vi "test-Coordinate-System-Test4.vi"() -> (3 "All tests passed":bool)   [LabVIEW 2019]
uses:
  <vilib>/Rock Robotics/WPI/ThirdParty/JAS_Junk/TrajLib/VI/CoordAxis_N.vi
  <vilib>/Rock Robotics/WPI/ThirdParty/JAS_Junk/TrajLib/VI/CoordSystem_New.vi
  <vilib>/Rock Robotics/WPI/ThirdParty/JAS_Junk/TrajLib/VI/CoordAxis_E.vi
  <vilib>/Rock Robotics/WPI/ThirdParty/JAS_Junk/TrajLib/VI/CoordAxis_D.vi
  <vilib>/Rock Robotics/WPI/ThirdParty/JAS_Junk/TrajLib/Conv_Deg_Radians.vi
  <vilib>/Rock Robotics/WPI/ThirdParty/JAS_Junk/TrajLib/VI/Quaternion_New.vi
  <vilib>/Rock Robotics/WPI/ThirdParty/JAS_Junk/TrajLib/VI/Translation3d_Create.vi
  <vilib>/Rock Robotics/WPI/ThirdParty/JAS_Junk/TrajLib/VI/Pose3d_New_Trans3dRot3d.vi
  <vilib>/Rock Robotics/WPI/ThirdParty/JAS_Junk/TrajLib/VI/CoordAxis_New.vi
  <vilib>/Rock Robotics/WPI/ThirdParty/JAS_Junk/TrajLib/MatBuilder_Create.vi
  <vilib>/Rock Robotics/WPI/ThirdParty/JAS_Junk/TrajLib/Matrix_AssignBlock.vi
  <vilib>/Rock Robotics/WPI/ThirdParty/JAS_Junk/TrajLib/VI/Rotation3D_Create_RotMatrix.vi
  <vilib>/Rock Robotics/WPI/ThirdParty/JAS_Junk/TrajLib/MatrixHelper_CoerceSize.vi
  <vilib>/Rock Robotics/WPI/ThirdParty/JAS_Junk/TrajLib/VI/Rotation3d_Create_Quaternion.vi
  <vilib>/Rock Robotics/WPI/ThirdParty/JAS_Junk/TrajLib/Matrix_Transpose.vi
  <vilib>/Analysis/baseanly.llb/A x B.vi
  <vilib>/Analysis/baseanly.llb/Real A x B.vi
  <vilib>/Rock Robotics/WPI/ThirdParty/JAS_Junk/TrajLib/Matrix_Ident.vi
  <vilib>/Rock Robotics/WPI/ThirdParty/JAS_Junk/TrajLib/Matrix_IsEqual.vi
  <vilib>/Analysis/baseanly.llb/Determinant.vi
  <vilib>/Analysis/baseanly.llb/Real Determinant.vi
  <vilib>/Rock Robotics/WPI/ThirdParty/JAS_Junk/TrajLib/VI/Quaternion_Normalize.vi
  <vilib>/Rock Robotics/WPI/ThirdParty/JAS_Junk/TrajLib/VI/Quaternion_New_Default.vi
  <vilib>/Analysis/Matrix/Numeric/Conversions/Array To Matrix.vi
  <vilib>/Analysis/Matrix/Numeric/Conversions/Array To Matrix - RA.vi
  <vilib>/Analysis/7linalg.llb/Create Special Matrix.vi
  <vilib>/Analysis/7linalg.llb/Create Special Real Matrix.vi
  <vilib>/Rock Robotics/WPI/ThirdParty/JAS_Junk/TrajLib/Trajectory_Library.lvlib
panel:
  out "Test 4":bool
  out "Test 3":bool
  out "Test 2":bool
  out "Test 1":bool
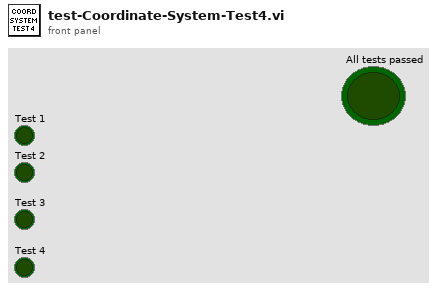
[diagram p1: front panel]
types:
  T1 = typedef "Trajectory_Library.lvlib/ROTATION3D.ctl" = cluster{"Q_quaternion":T2}
  T2 = typedef "Trajectory_Library.lvlib/QUATERNION.ctl" = cluster{"R":dbl, "V":dbl[]}
  T3 = typedef "Trajectory_Library.lvlib/POSE3D.ctl" = cluster{"Translation3d":T4, "Rotation3d":T1}
  T4 = typedef "Trajectory_Library.lvlib/TRANSLATION3D.ctl" = cluster{"X":dbl, "Y":dbl, "Z":dbl}
  T5 = typedef "Trajectory_Library.lvlib/COORDINATE_SYSTEM.ctl" = cluster{"Rotation":T1}
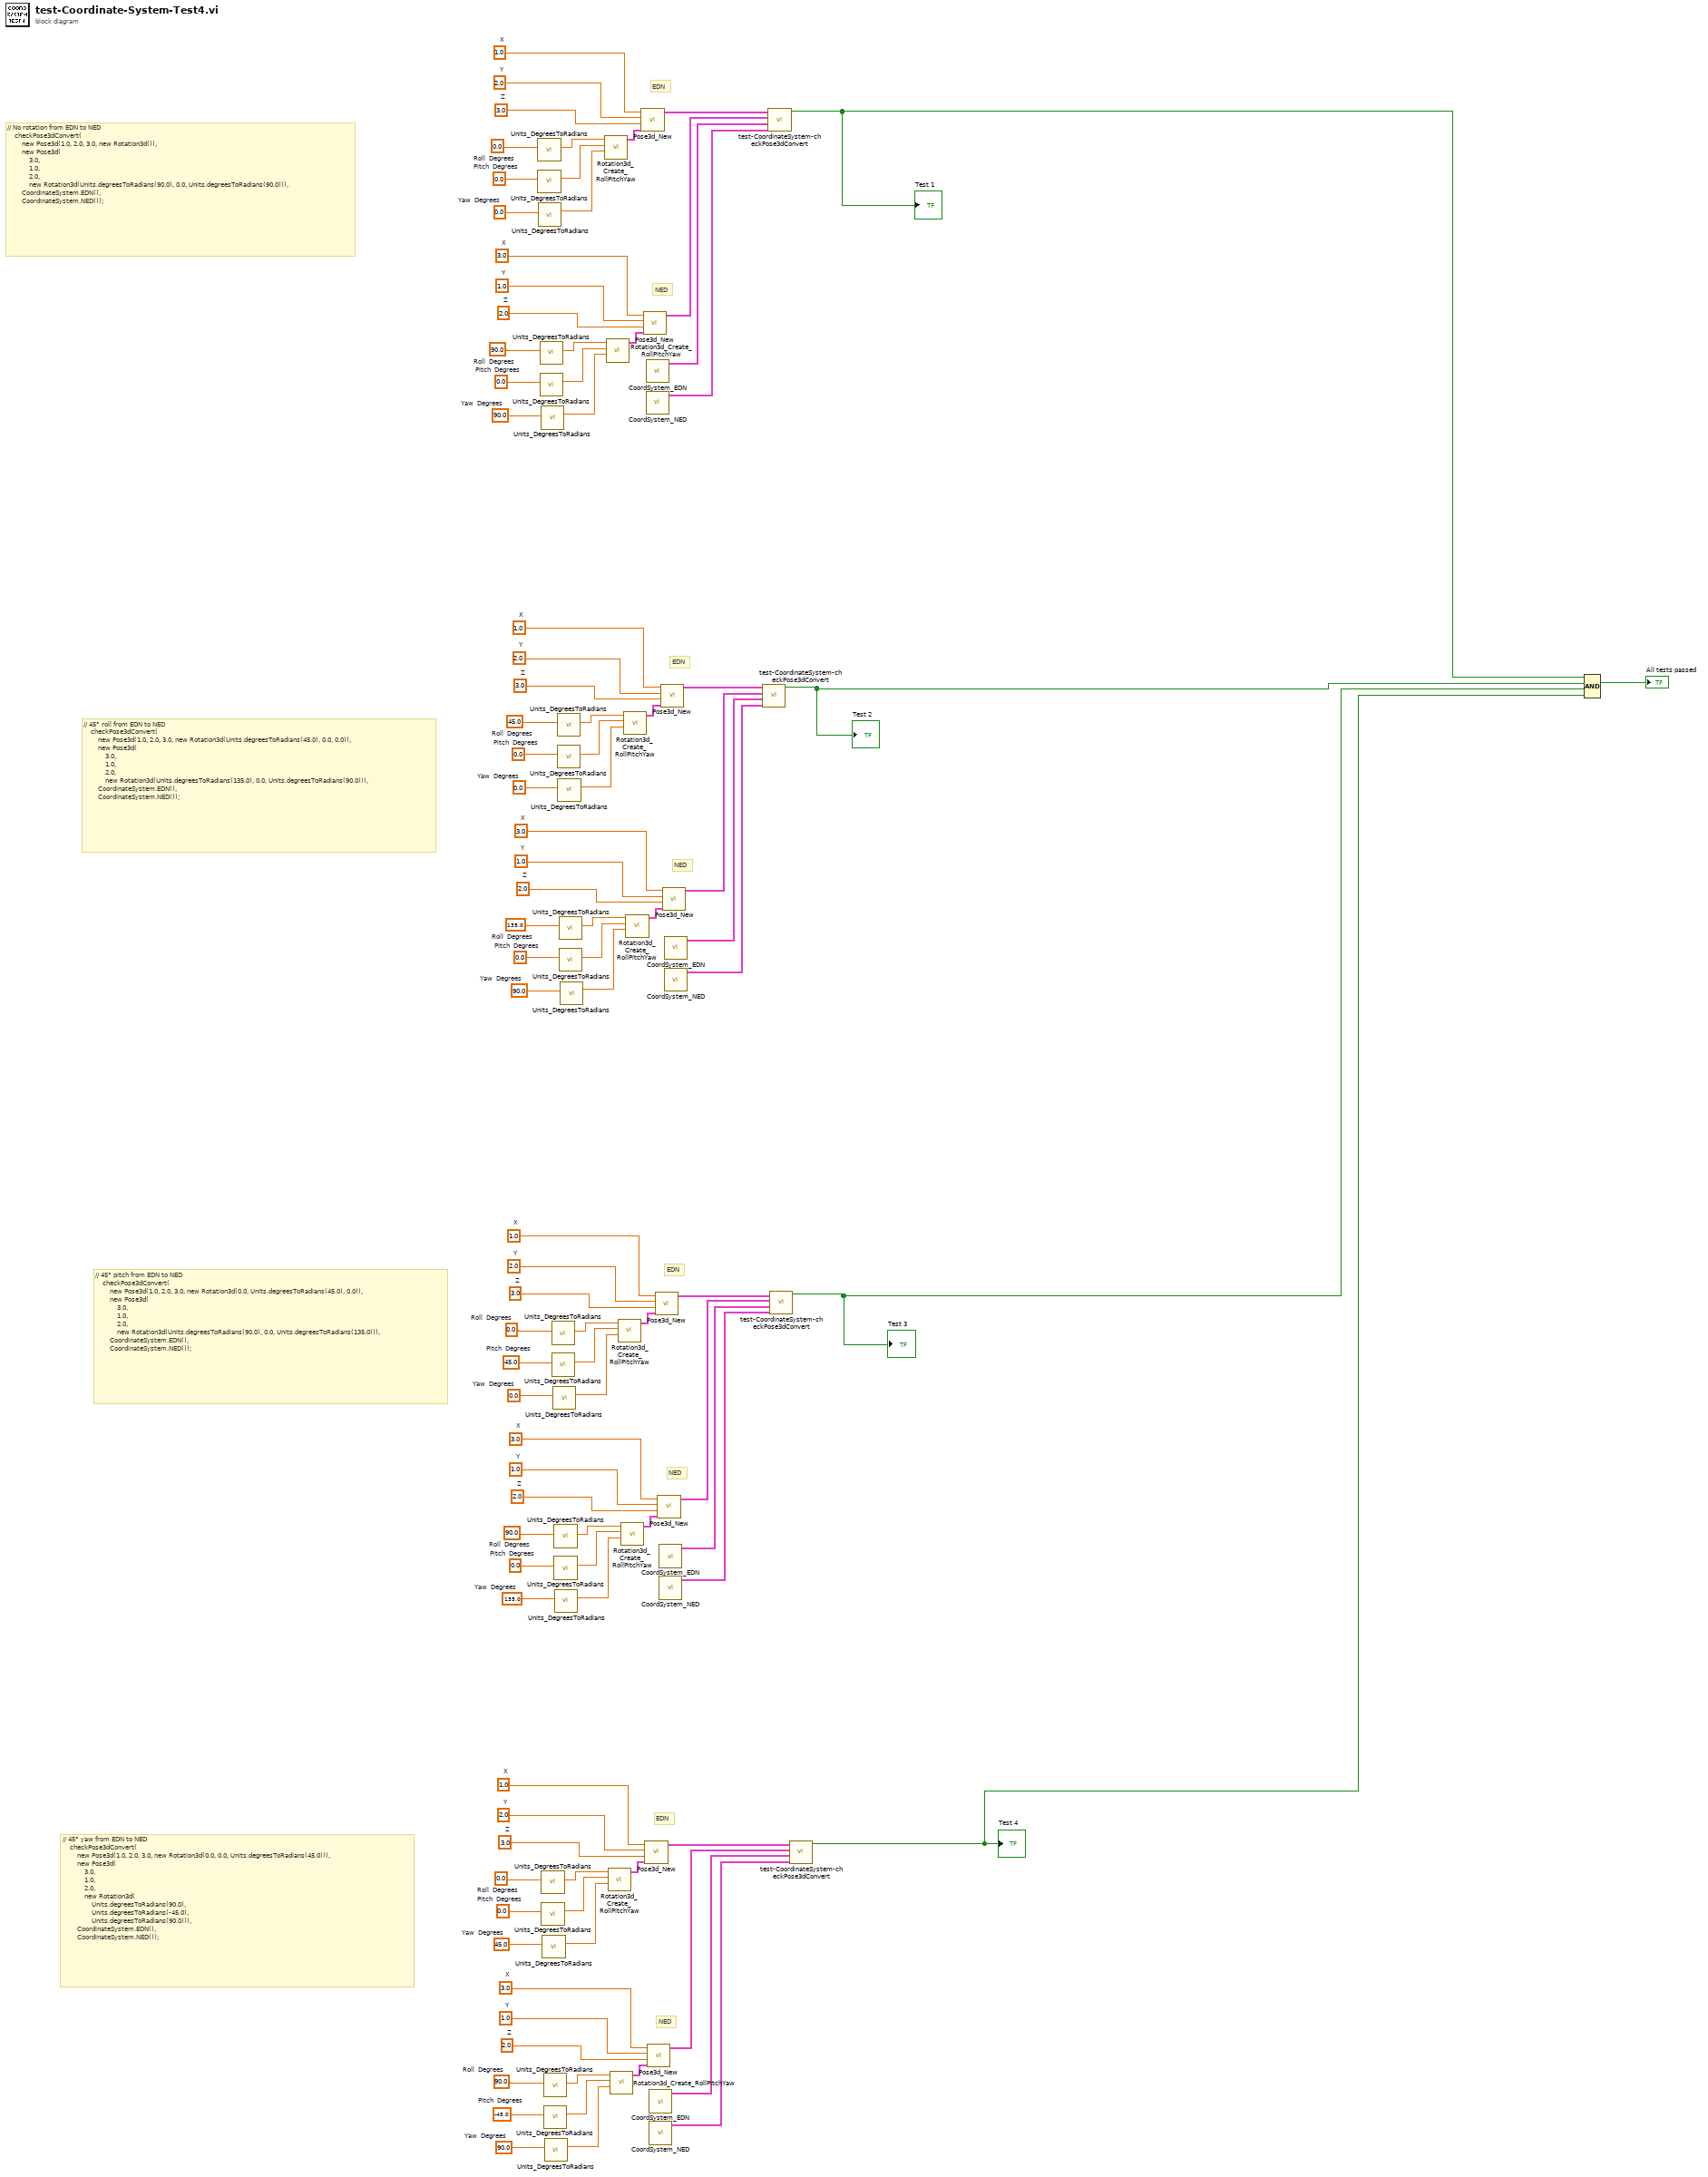
[diagram p0: block diagram]
diagram:
  w29 = 3.0  # X
  w28 = 1.0  # Y
  w27 = 2.0  # Z
  w21 = 90.0  # Roll  Degrees
  w22 = -45.0  # Pitch  Degrees
  w23 = 90.0  # Yaw  Degrees
  w39 = 1.0  # X
  w38 = 2.0  # Y
  w37 = 3.0  # Z
  w31 = 0.0  # Roll  Degrees
  w32 = 0.0  # Pitch  Degrees
  w33 = 45.0  # Yaw  Degrees
  w49 = 3.0  # X
  w48 = 1.0  # Y
  w47 = 2.0  # Z
  w41 = 90.0  # Roll  Degrees
  w42 = 0.0  # Pitch  Degrees
  w43 = 135.0  # Yaw  Degrees
  w59 = 1.0  # X
  w58 = 2.0  # Y
  w57 = 3.0  # Z
  w51 = 0.0  # Roll  Degrees
  w52 = 45.0  # Pitch  Degrees
  w53 = 0.0  # Yaw  Degrees
  w69 = 3.0  # X
  w68 = 1.0  # Y
  w67 = 2.0  # Z
  w61 = 135.0  # Roll  Degrees
  w62 = 0.0  # Pitch  Degrees
  w63 = 90.0  # Yaw  Degrees
  w79 = 1.0  # X
  w78 = 2.0  # Y
  w77 = 3.0  # Z
  w71 = 45.0  # Roll  Degrees
  w72 = 0.0  # Pitch  Degrees
  w73 = 0.0  # Yaw  Degrees
  w90 = 3.0  # X
  w89 = 1.0  # Y
  w88 = 2.0  # Z
  w82 = 90.0  # Roll  Degrees
  w83 = 0.0  # Pitch  Degrees
  w84 = 90.0  # Yaw  Degrees
  w100 = 1.0  # X
  w99 = 2.0  # Y
  w98 = 3.0  # Z
  w92 = 0.0  # Roll  Degrees
  w93 = 0.0  # Pitch  Degrees
  w94 = 0.0  # Yaw  Degrees
  # "// 45° roll from EDN to NED\n    checkPose3dConvert(\n        new Pose3d(1.0, 2.0, 3.0, new Rotation3d(Units.degreesToRadians(45.0), 0.0, 0.0)),\n        new Pose3d(\n            3.0,\n            1.0,\n            2.0,\n            new Rotation3d(Units.degreesToRadians(135.0), 0.0, Units.degreesToRadians(90.0))),\n        CoordinateSystem.EDN(),\n        CoordinateSystem.NED());"
  # "// No rotation from EDN to NED\n    checkPose3dConvert(\n        new Pose3d(1.0, 2.0, 3.0, new Rotation3d()),\n        new Pose3d(\n            3.0,\n            1.0,\n            2.0,\n            new Rotation3d(Units.degreesToRadians(90.0), 0.0, Units.degreesToRadians(90.0))),\n        CoordinateSystem.EDN(),\n        CoordinateSystem.NED());"
  # "// 45° yaw from EDN to NED\n    checkPose3dConvert(\n        new Pose3d(1.0, 2.0, 3.0, new Rotation3d(0.0, 0.0, Units.degreesToRadians(45.0))),\n        new Pose3d(\n            3.0,\n            1.0,\n            2.0,\n            new Rotation3d(\n                Units.degreesToRadians(90.0),\n                Units.degreesToRadians(-45.0),\n                Units.degreesToRadians(90.0))),\n        CoordinateSystem.EDN(),\n        CoordinateSystem.NED());"
  # "NED"
  # "EDN"
  # "NED"
  # "EDN"
  # "// 45° pitch from EDN to NED\n    checkPose3dConvert(\n        new Pose3d(1.0, 2.0, 3.0, new Rotation3d(0.0, Units.degreesToRadians(45.0), 0.0)),\n        new Pose3d(\n            3.0,\n            1.0,\n            2.0,\n            new Rotation3d(Units.degreesToRadians(90.0), 0.0, Units.degreesToRadians(135.0))),\n        CoordinateSystem.EDN(),\n        CoordinateSystem.NED());"
  # "NED"
  # "EDN"
  # "NED"
  # "EDN"
  n1 = call <vilib>:"Units_DegreesToRadians.vi"("Degrees"=w92) -> ("Radians"=w95:dbl)  [unwired: 10 in]
  n2 = call <vilib>:"Units_DegreesToRadians.vi"("Degrees"=w93) -> ("Radians"=w96:dbl)  [unwired: 10 in]
  n3 = call <vilib>:"Units_DegreesToRadians.vi"("Degrees"=w94) -> ("Radians"=w97:dbl)  [unwired: 10 in]
  n4 = call <vilib>:"Units_DegreesToRadians.vi"("Degrees"=w82) -> ("Radians"=w85:dbl)  [unwired: 10 in]
  n5 = call <vilib>:"Units_DegreesToRadians.vi"("Degrees"=w83) -> ("Radians"=w86:dbl)  [unwired: 10 in]
  n6 = call <vilib>:"Units_DegreesToRadians.vi"("Degrees"=w84) -> ("Radians"=w87:dbl)  [unwired: 10 in]
  n7 = call <vilib>:"Units_DegreesToRadians.vi"("Degrees"=w31) -> ("Radians"=w34:dbl)  [unwired: 10 in]
  n8 = call <vilib>:"Units_DegreesToRadians.vi"("Degrees"=w32) -> ("Radians"=w35:dbl)  [unwired: 10 in]
  n9 = call <vilib>:"Units_DegreesToRadians.vi"("Degrees"=w33) -> ("Radians"=w36:dbl)  [unwired: 10 in]
  n10 = call <vilib>:"Units_DegreesToRadians.vi"("Degrees"=w21) -> ("Radians"=w24:dbl)  [unwired: 10 in]
  n11 = call <vilib>:"Units_DegreesToRadians.vi"("Degrees"=w22) -> ("Radians"=w25:dbl)  [unwired: 10 in]
  n12 = call <vilib>:"Units_DegreesToRadians.vi"("Degrees"=w23) -> ("Radians"=w26:dbl)  [unwired: 10 in]
  n13 = call <vilib>:"Units_DegreesToRadians.vi"("Degrees"=w51) -> ("Radians"=w54:dbl)  [unwired: 10 in]
  n14 = call <vilib>:"Units_DegreesToRadians.vi"("Degrees"=w52) -> ("Radians"=w55:dbl)  [unwired: 10 in]
  n15 = call <vilib>:"Units_DegreesToRadians.vi"("Degrees"=w53) -> ("Radians"=w56:dbl)  [unwired: 10 in]
  n16 = call <vilib>:"Units_DegreesToRadians.vi"("Degrees"=w41) -> ("Radians"=w44:dbl)  [unwired: 10 in]
  n17 = call <vilib>:"Units_DegreesToRadians.vi"("Degrees"=w42) -> ("Radians"=w45:dbl)  [unwired: 10 in]
  n18 = call <vilib>:"Units_DegreesToRadians.vi"("Degrees"=w43) -> ("Radians"=w46:dbl)  [unwired: 10 in]
  n19 = call <vilib>:"Units_DegreesToRadians.vi"("Degrees"=w71) -> ("Radians"=w74:dbl)  [unwired: 10 in]
  n20 = call <vilib>:"Units_DegreesToRadians.vi"("Degrees"=w72) -> ("Radians"=w75:dbl)  [unwired: 10 in]
  n21 = call <vilib>:"Units_DegreesToRadians.vi"("Degrees"=w73) -> ("Radians"=w76:dbl)  [unwired: 10 in]
  n22 = call <vilib>:"Units_DegreesToRadians.vi"("Degrees"=w61) -> ("Radians"=w64:dbl)  [unwired: 10 in]
  n23 = call <vilib>:"Units_DegreesToRadians.vi"("Degrees"=w62) -> ("Radians"=w65:dbl)  [unwired: 10 in]
  n24 = call <vilib>:"Units_DegreesToRadians.vi"("Degrees"=w63) -> ("Radians"=w66:dbl)  [unwired: 10 in]
  n25 = call <vilib>:"Rotation3d_Create_RollPitchYaw.vi"("Yaw"=w97, "Pitch"=w96, "Roll"=w95) -> ("Rotation3d"=w101:T1)  [unwired: 8 in]
  n26 = call <vilib>:"Rotation3d_Create_RollPitchYaw.vi"("Yaw"=w87, "Pitch"=w86, "Roll"=w85) -> ("Rotation3d"=w91:T1)  [unwired: 8 in]
  n27 = call <vilib>:"Rotation3d_Create_RollPitchYaw.vi"("Yaw"=w36, "Pitch"=w35, "Roll"=w34) -> ("Rotation3d"=w40:T1)  [unwired: 8 in]
  n28 = call <vilib>:"Rotation3d_Create_RollPitchYaw.vi"("Yaw"=w26, "Pitch"=w25, "Roll"=w24) -> ("Rotation3d"=w30:T1)  [unwired: 8 in]
  n29 = call <vilib>:"Rotation3d_Create_RollPitchYaw.vi"("Yaw"=w56, "Pitch"=w55, "Roll"=w54) -> ("Rotation3d"=w60:T1)  [unwired: 8 in]
  n30 = call <vilib>:"Rotation3d_Create_RollPitchYaw.vi"("Yaw"=w46, "Pitch"=w45, "Roll"=w44) -> ("Rotation3d"=w50:T1)  [unwired: 8 in]
  n31 = call <vilib>:"Rotation3d_Create_RollPitchYaw.vi"("Yaw"=w76, "Pitch"=w75, "Roll"=w74) -> ("Rotation3d"=w80:T1)  [unwired: 8 in]
  n32 = call <vilib>:"Rotation3d_Create_RollPitchYaw.vi"("Yaw"=w66, "Pitch"=w65, "Roll"=w64) -> ("Rotation3d"=w70:T1)  [unwired: 8 in]
  n33 = call <vilib>:"Pose3d_New.vi"("Rotation3d"=w101, "z"=w98, "Y"=w99, "X"=w100) -> ("out Pose3d"=w5:T3)  [unwired: 7 in]
  n34 = call <vilib>:"Pose3d_New.vi"("Rotation3d"=w91, "z"=w88, "Y"=w89, "X"=w90) -> ("out Pose3d"=w4:T3)  [unwired: 7 in]
  n35 = call <vilib>:"Pose3d_New.vi"("Rotation3d"=w40, "z"=w37, "Y"=w38, "X"=w39) -> ("out Pose3d"=w20:T3)  [unwired: 7 in]
  n36 = call <vilib>:"CoordSystem_EDN.vi"() -> ("out Coordinate System"=w3:T5)  [unwired: 10 in, 1 out]
  n37 = call <vilib>:"CoordSystem_NED.vi"() -> ("out Coordinate System"=w2:T5)  [unwired: 10 in, 1 out]
  n38 = call <vilib>:"Pose3d_New.vi"("Rotation3d"=w30, "z"=w27, "Y"=w28, "X"=w29) -> ("out Pose3d"=w19:T3)  [unwired: 7 in]
  n39 = call <vilib>:"CoordSystem_EDN.vi"() -> ("out Coordinate System"=w18:T5)  [unwired: 10 in, 1 out]
  n40 = call <vilib>:"CoordSystem_NED.vi"() -> ("out Coordinate System"=w17:T5)  [unwired: 10 in, 1 out]
  n41 = call <vilib>:"Pose3d_New.vi"("Rotation3d"=w60, "z"=w57, "Y"=w58, "X"=w59) -> ("out Pose3d"=w15:T3)  [unwired: 7 in]
  n42 = call <vilib>:"Pose3d_New.vi"("Rotation3d"=w50, "z"=w47, "Y"=w48, "X"=w49) -> ("out Pose3d"=w14:T3)  [unwired: 7 in]
  n43 = call <vilib>:"CoordSystem_EDN.vi"() -> ("out Coordinate System"=w12:T5)  [unwired: 10 in, 1 out]
  n44 = call <vilib>:"CoordSystem_NED.vi"() -> ("out Coordinate System"=w13:T5)  [unwired: 10 in, 1 out]
  n45 = call <vilib>:"Pose3d_New.vi"("Rotation3d"=w80, "z"=w77, "Y"=w78, "X"=w79) -> ("out Pose3d"=w10:T3)  [unwired: 7 in]
  n46 = call <vilib>:"Pose3d_New.vi"("Rotation3d"=w70, "z"=w67, "Y"=w68, "X"=w69) -> ("out Pose3d"=w9:T3)  [unwired: 7 in]
  n47 = call <vilib>:"CoordSystem_EDN.vi"() -> ("out Coordinate System"=w8:T5)  [unwired: 10 in, 1 out]
  n48 = call <vilib>:"CoordSystem_NED.vi"() -> ("out Coordinate System"=w7:T5)  [unwired: 10 in, 1 out]
  n49 = call "test-CoordinateSystem-checkPose3dConvert.vi"("COORDINATE_SYSTEM_TO"=w7, "COORDINATE_SYSTEM_FROM"=w8, "Pose3D_TO"=w9, "Pose3d_FROM"=w10) -> ("All tests passed"=w6:bool)  [unwired: 7 in]
  "Test 2" <- w6
  n50 = call "test-CoordinateSystem-checkPose3dConvert.vi"("COORDINATE_SYSTEM_TO"=w2, "COORDINATE_SYSTEM_FROM"=w3, "Pose3D_TO"=w4, "Pose3d_FROM"=w5) -> ("All tests passed"=w1:bool)  [unwired: 7 in]
  "Test 1" <- w1
  n51 = call "test-CoordinateSystem-checkPose3dConvert.vi"("COORDINATE_SYSTEM_TO"=w13, "COORDINATE_SYSTEM_FROM"=w12, "Pose3D_TO"=w14, "Pose3d_FROM"=w15) -> ("All tests passed"=w11:bool)  [unwired: 7 in]
  "Test 3" <- w11
  n52 = call "test-CoordinateSystem-checkPose3dConvert.vi"("COORDINATE_SYSTEM_TO"=w17, "COORDINATE_SYSTEM_FROM"=w18, "Pose3D_TO"=w19, "Pose3d_FROM"=w20) -> ("All tests passed"=w16:bool)  [unwired: 7 in]
  "Test 4" <- w16
  n53 = Compound Arithmetic op=AND(w1, w6, w11, w16) -> (→"All tests passed":bool)
